vi "URAPI_WhileStart.vi"(0 "Variable In":string, 1 "Compare to":string="10", 3 "URAPI Script":T1={"Script"="", "Whiles"=[], "Ifs"=[], "Supress Err"=TRUE, "Errors"=""}, 4 "Comparison":enum16{">", "<", ">=", "<=", "=", "!="}(ring)=enum."<") -> (2 "variable":string="count0", 5 "URAPI Script Out":T1={"Script"="count0=0\n//while0 conditional \nwhileLand0:\nIF ~(voltage > 100) goto endwhile0\n", "Whiles"=[0], "Ifs"=[], "Supress Err"=TRUE, "Errors"=""})   [LabVIEW 2012]
doc: "Commmences a while loop. The condition is based on a comparison of \"Variable in\" against \"Compare to\", using the specified \"Comparison\" constant. This loop will continue to execute until this comparison is not true. \nNote: requires Loop end VI."
uses:
  <userlib>/BotSpeak/VIs/Direct/URAPI_Control.ctl
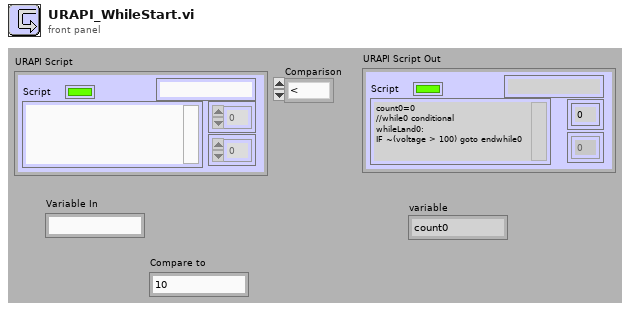
[diagram p1: front panel]
types:
  T1 = typedef "URAPI_Control.ctl" = cluster{"Script":string, "Whiles":u8[], "Ifs":u8[], "Supress Err":bool, "Errors":string}
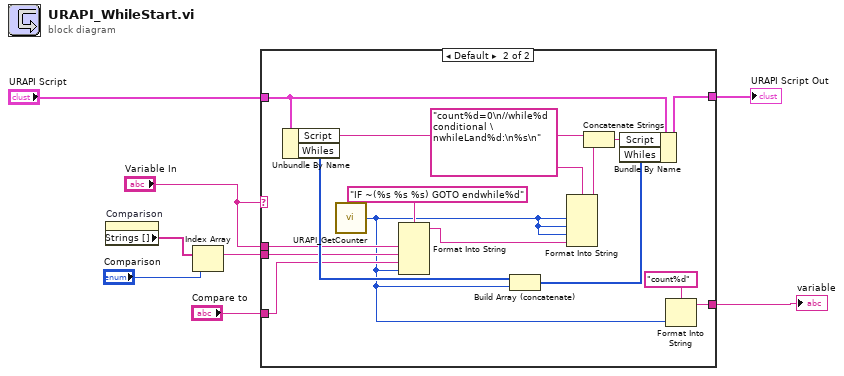
[diagram p0: block diagram]
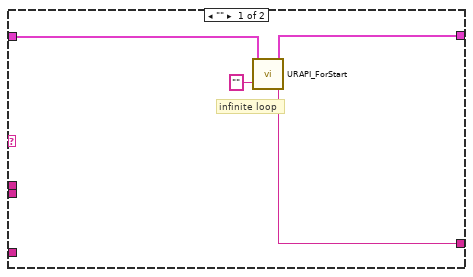
[diagram p2: hidden frame]
diagram:
  n1 = property on="Comparison" class="Enum (strict)"() -> ("Strings []"=w6:string[])  [unwired: 2 in, 2 out]
  n2 = Index Array(array=w6, index="Comparison") -> (element=w4:string)
  n3 = case shown="Default" "Variable In" {
    tunnel: [w11 w28] -> w8
    tunnel: "URAPI Script" -> [w12 w27]
    tunnel: "Variable In" -> [_ w19]
    tunnel: w4 -> [_ w18]
    tunnel: "Compare to" -> [_ w17]
    tunnel: [w10 w13] -> w1
    frame "" {
      # "infinite loop"
      n4 = call <userlib>:"URAPI_ForStart.vi"("Iterations"="", "URAPI Script"=w12) -> ("variable"=w10:string, "URAPI Script Out"=w11:T1)  [unwired: 2 in]
    }
    frame Default {
      n5 = Unbundle By Name(w27) -> ("Script"=w23:string, "Whiles"=w22:u8[])
      n6 = call <userlib>:"URAPI_GetCounter.vi"() -> ("Numeric"=w14:u16)  [unwired: 1 in]
      n7 = Format Into String(format string="IF ~(%s %s %s) GOTO endwhile%d" ("string"), w19, w18, w17, w14) -> (resulting string=w16:string)  [unwired: 2 in, 1 out]
      n8 = Build Array (concatenate)(w22, w14) -> (w21:u16[])
      n9 = Format Into String(format string="count%d=0\n//while%d conditional \nwhileLand%d:\n%s\n" ("string"), w14, w14, w14, w16) -> (resulting string=w24:string)  [unwired: 2 in, 1 out]
      n10 = Concatenate Strings(w23, w24) -> (w26:string)
      n11 = Bundle By Name(cluster=w27, "Script"=w26, "Whiles"=w21) -> (w28:T1)
      n12 = Format Into String(format string="count%d", w14) -> (resulting string=w13:string)  [unwired: 2 in, 1 out]
    }
  }
  "URAPI Script Out" <- w8
  "variable" <- w1
